vi "Determine If Belongs In Sector and Accumulate.vi"(6 "Left Sector Parameters":T3, 7 "Right Sector Parameters":T3, 8 "error in (no error)":errorcluster, 9 "Midpoint of Image":dbl, 10 "Starting Y Location":i32, 11 "Image Data":u8[][](array[numeric])) -> (0 "error out":errorcluster, 2 "Canceled?":bool, 3 "[Accumulated Sectors]":T2[](array[typedef]))   [LabVIEW 2013]
uses:
  FPGA/Sector/Accumulate/Sector Parameter Cluster.ctl
  FPGA/Sector/Accumulate/Accumulated Sector Cluster.ctl
  Test Compiliation/Test Sector Cluster.ctl
panel:
  out "Pixel Sectors":T1[](array[typedef])
  in  "Cancel Button":bool
  out "Progress":u16(slide) scale=0.0..788.0
  # "Calculating Average Sector Background ..."
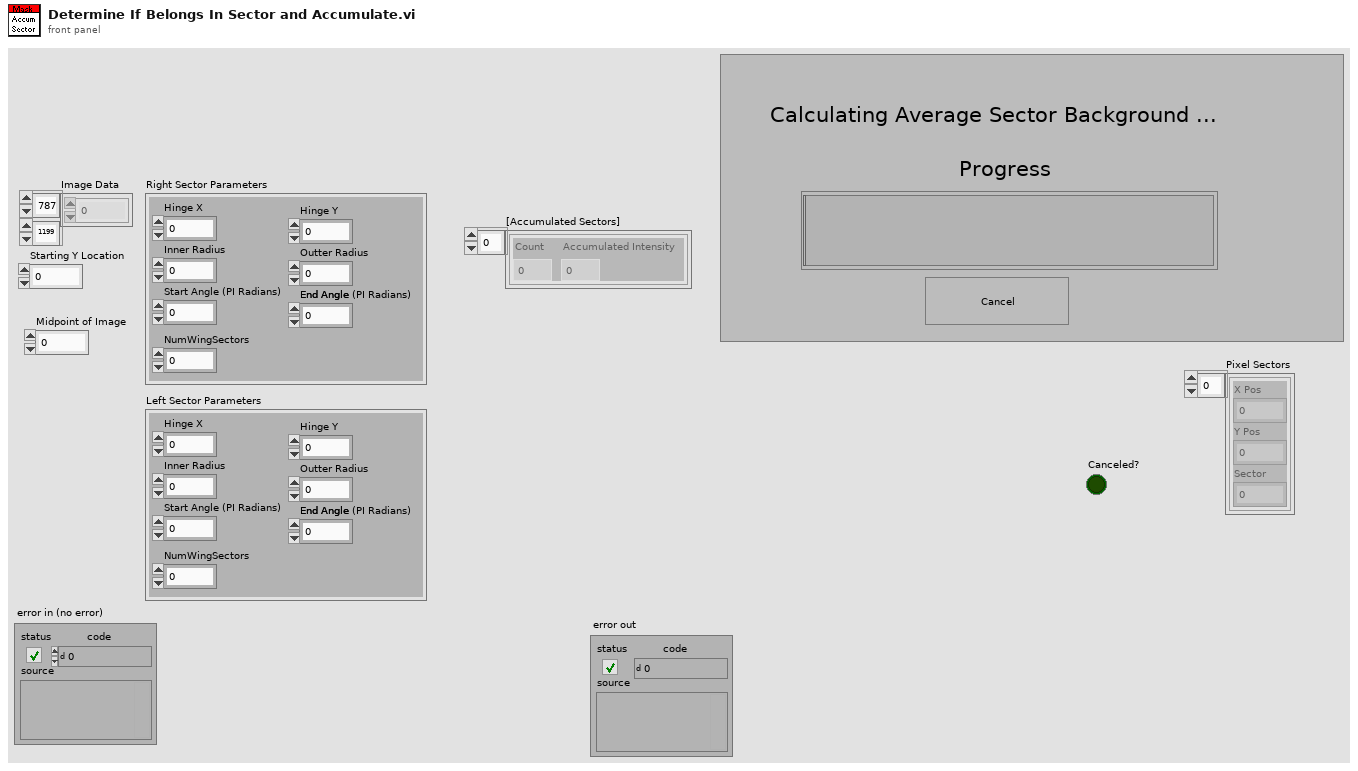
[diagram p1: front panel]
types:
  T1 = typedef "Test Sector Cluster.ctl" = cluster{"X Pos":u16, "Y Pos":u16, "Sector":u8}
  T2 = typedef "Accumulated Sector Cluster.ctl" = cluster{"Accumulated Intensity":u32, "Count":u16}
  T3 = typedef "Sector Parameter Cluster.ctl" = cluster{"Start Angle":fxp<+/-,17,2>, "End Angle":fxp<+/-,17,2>, "Inner Radius":u16, "Outter Radius":u16, "Hinge X":u16, "Hinge Y":u16, "NumWingSectors":u8}
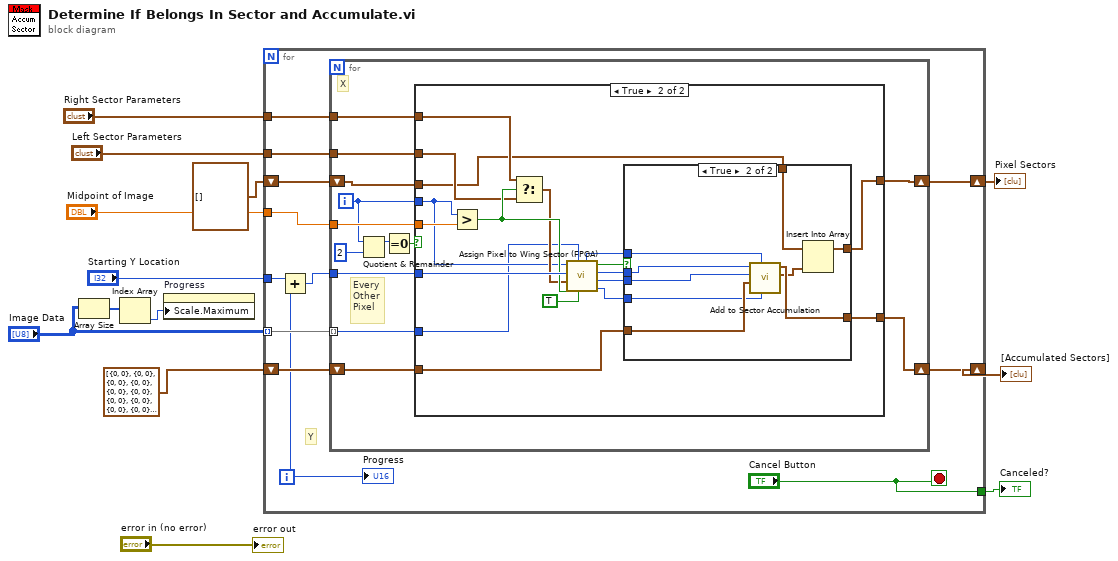
[diagram p0: block diagram]
diagram:
  n1 = Array Size(array="Image Data") -> (size(s)=w5:i32[])
  n2 = Index Array(array=w5) -> (element=w4:i32)  [unwired: 1 in]
  n3 = property on="Progress" class="Slide (strict)"("Scale.Maximum"=w4) -> ()  [unwired: 2 in, 2 out]
  n4 = for {
    tunnel: "Image Data" -> [w25] mode=indexing
    tunnel: "Midpoint of Image" -> [w24]
    tunnel: "Right Sector Parameters" -> [w23]
    tunnel: "Left Sector Parameters" -> [w22]
    shift-right: [w20] -> w8
    shift-left: T2[] [{"Accumulated Intensity"=0, "Count"=0}, {"Accumulated Intensity"=0, "Count"=0}, {"Accumulated Intensity"=0, "Count"=0}, {"Accumulated Intensity"=0, "Count"=0}, {"Accumulated Intensity"=0, "Count"=0}, {"Accumulated Intensity"=0, "Count"=0}, {"Accumulated Intensity"=0, "Count"=0}, {"Accumulated Intensity"=0, "Count"=0}, {"Accumulated Intensity"=0, "Count"=0}, {"Accumulated Intensity"=0, "Count"=0}, {"Accumulated Intensity"=0, "Count"=0}, {"Accumulated Intensity"=0, "Count"=0}, {"Accumulated Intensity"=0, "Count"=0}, {"Accumulated Intensity"=0, "Count"=0}, {"Accumulated Intensity"=0, "Count"=0}, {"Accumulated Intensity"=0, "Count"=0}, {"Accumulated Intensity"=0, "Count"=0}, {"Accumulated Intensity"=0, "Count"=0}, {"Accumulated Intensity"=0, "Count"=0}, {"Accumulated Intensity"=0, "Count"=0}, {"Accumulated Intensity"=0, "Count"=0}, {"Accumulated Intensity"=0, "Count"=0}, {"Accumulated Intensity"=0, "Count"=0}, {"Accumulated Intensity"=0, "Count"=0}, {"Accumulated Intensity"=0, "Count"=0}, {"Accumulated Intensity"=0, "Count"=0}, {"Accumulated Intensity"=0, "Count"=0}, {"Accumulated Intensity"=0, "Count"=0}, {"Accumulated Intensity"=0, "Count"=0}, {"Accumulated Intensity"=0, "Count"=0}, {"Accumulated Intensity"=0, "Count"=0}, {"Accumulated Intensity"=0, "Count"=0}] ("[Accumulated Sectors] Out") -> [w21]
    tunnel: "Starting Y Location" -> [w18]
    tunnel: ["Cancel Button"] -> w3
    shift-right: [w14] -> w1
    shift-left: T1[] [] ("array") -> [w15]
    i -> [w17]
    stop <- "Cancel Button" stop-if-true
    # "Y"
    n5 = Add(x=w18, y=w17) -> (x+y=w19:i32)
    n6 = for {
      tunnel: w25 -> [w34] mode=indexing
      tunnel: w19 -> [w38]
      tunnel: w24 -> [w37]
      tunnel: w23 -> [w36]
      tunnel: w22 -> [w35]
      shift-right: [w32] -> w20
      shift-left: w21 -> [w33]
      shift-right: [w26] -> w14
      shift-left: w15 -> [w27]
      i -> [w31]
      # "Every\nOther\nPixel"
      # "X"
      n7 = Quotient & Remainder(x=w31, y=2) -> (x-y*floor(x/y)=w29:i32)  [unwired: 1 out]
      n8 = Equal To 0?(x=w29) -> (x = 0?=w28:bool)
      n9 = case shown="True" w28 {
        tunnel: w38 -> [_ w58]
        tunnel: w37 -> [_ w57]
        tunnel: w36 -> [_ w55]
        tunnel: w35 -> [_ w54]
        tunnel: w31 -> [_ w52]
        tunnel: w34 -> [_ w51]
        tunnel: w33 -> [w40 w49]
        tunnel: [w40 w47] -> w32
        tunnel: w27 -> [w39 w45]
        tunnel: [w39 w44] -> w26
        frame False {
        }
        frame True {
          n10 = Greater?(x=w52, y=w57) -> (0:w56:bool)
          n11 = Select(t=w55, s=w56, f=w54) -> (s? t:f=w53:T3)
          n12 = call "Assign Pixel to Wing Sector (FPGA).vi"("Valid Data?"=TRUE, "Pixel Intensity In"=w51, "Right Wing?"=w56, "Sector Parameters"=w53, "Pixel Y"=w58, "Pixel X"=w52) -> ("Y Pixel Out"=w41:u16, "Pixel Intensity Out"=w46:u8, "sector #"=w48:u8, "output valid"=w50:bool, "X Pixel Out"=w42:u16)  [unwired: 1 in]
          n13 = case shown="True" w50 {
            tunnel: w49 -> [w60 w67]
            tunnel: w48 -> [_ w69]
            tunnel: [w60 w66] -> w47
            tunnel: w46 -> [_ w68]
            tunnel: w45 -> [w59 w63]
            tunnel: [w59 w65] -> w44
            tunnel: w42 -> [_ w62]
            tunnel: w41 -> [_ w61]
            frame False {
            }
            frame True {
              n14 = call "Add to Sector Accumulation.vi"("Pixel y"=w61, "Pixel x"=w62, "[Accumulated Sectors] In"=w67, "Pixel Intensity"=w68, "Sector ID"=w69) -> ("Sector Pixel"=w64:T1, "[Accumulated Sectors] Out"=w66:T2[])  [unwired: 5 in]
              n15 = Insert Into Array(array=w63, new element=w64) -> (w65:T1[])  [unwired: 1 in]
            }
          }
        }
      }
    }
    "Progress" <- w17
  }
  "[Accumulated Sectors]" <- w8
  "Canceled?" <- w3
  "Pixel Sectors" <- w1
  "error out" <- "error in (no error)"
